vi "Calibration INI tester.vi"() -> ()   [LabVIEW 2020]
uses:
  Typedefs/Calibration config.ctl
  Typedefs/Objective Config.ctl
  Typedefs/Prechirper Cal Config.ctl
  Typedefs/PreChirper constants.ctl
panel:
  in  "Save to":path
  in  "Load from":path
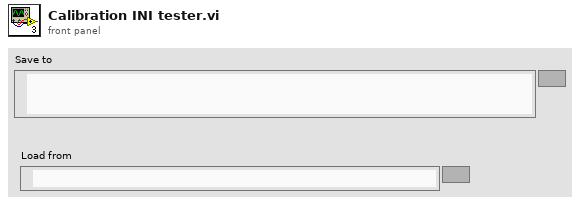
[diagram p1: front panel]
types:
  T1 = typedef "PreChirper constants.ctl" = cluster{"a 1":i32, "b 1":i32, "c 1":i32, "a 2":i32, "b 2":i32, "c 2":i32, "lmin":i32, "lmax":i32}
  T2 = typedef "Prechirper Cal Config.ctl" = cluster{"Wavelength":i32, "Prism 1":i32, "Prism 2":i32}
  T3 = typedef "Objective Config.ctl" = cluster{"Name":string, "Sum X":dbl, "Sum Y":dbl, "Diff X":dbl, "Diff Y":dbl, "Distortion Correction":dbl, "Z_norm to um_scaling":dbl, "X_norm to um_scaling":dbl, "Calibrated Wavelength":dbl}
  T4 = typedef "Calibration config.ctl" = cluster{"Current Objective":string, "Objective Settings":T3[], "PreChirper Values Preset ?":bool, "PreChirper Settings":T2[], "PreChirper Constants":T1}
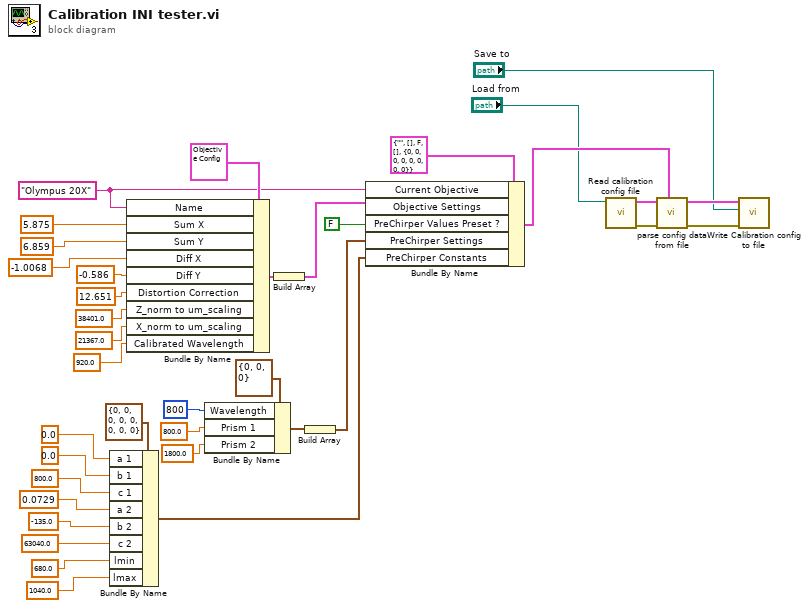
[diagram p0: block diagram]
diagram:
  w35 = "Olympus 20X" ("Current Objective")
  n1 = Bundle By Name(cluster=T1 {"a 1"=0, "b 1"=0, "c 1"=0, "a 2"=0, "b 2"=0, "c 2"=0, "lmin"=0, "lmax"=0} ("Prechirper Constants"), "a 1"=0.0, "b 1"=0.0, "c 1"=800.0, "a 2"=0.0729, "b 2"=-135.0, "c 2"=63040.0, "lmin"=680.0, "lmax"=1040.0) -> (w10:T1)
  n2 = Bundle By Name(cluster=T3 {"Name"="", "Sum X"=0.0, "Sum Y"=0.0, "Diff X"=0.0, "Diff Y"=0.0, "Distortion Correction"=0.0, "Z_norm to um_scaling"=0.0, "X_norm to um_scaling"=0.0, "Calibrated Wavelength"=0.0} ("Objective HW Settings"), "Name"=w35, "Sum X"=5.875, "Sum Y"=6.859, "Diff X"=-1.0068 ("Sum Y"), "Diff Y"=-0.586 ("Sum Y"), "Distortion Correction"=12.651 ("Sum Y"), "Z_norm to um_scaling"=38401.0 ("Sum Y"), "X_norm to um_scaling"=21367.0 ("Sum Y"), "Calibrated Wavelength"=920.0) -> (w26:T3)
  n3 = Bundle By Name(cluster=T2 {"Wavelength"=0, "Prism 1"=0, "Prism 2"=0} ("Prechirper Config"), "Wavelength"=800, "Prism 1"=800.0, "Prism 2"=1800.0) -> (w22:T2)
  n4 = Build Array(w26) -> (w25:T3[])
  n5 = Build Array(w22) -> (w9:T2[])
  n6 = Bundle By Name(cluster=T4 {"Current Objective"="", "Objective Settings"=[], "PreChirper Values Preset ?"=FALSE, "PreChirper Settings"=[], "PreChirper Constants"={"a 1"=0, "b 1"=0, "c 1"=0, "a 2"=0, "b 2"=0, "c 2"=0, "lmin"=0, "lmax"=0}} ("Config cluster IN"), "Current Objective"=w35, "Objective Settings"=w25, "PreChirper Values Preset ?"=FALSE, "PreChirper Settings"=w9, "PreChirper Constants"=w10) -> (w5:T4)
  n7 = call "Read calibration config file.vi"("configuration file path"="Load from") -> ("error out"=w6:errorcluster, "Array"=w7:cluster{"String":string, string[]}[])  [unwired: 9 in]
  n8 = call "parse config data from file.vi"("Calibration Config"=w5, "Error in"=w6, "Array"=w7) -> ("Error out"=w3:errorcluster, "Config cluster"=w2:T4)  [unwired: 7 in]
  n9 = call "Write Calibration config to file.vi"("error in (no error)"=w3, "configuration file path"="Save to", "Calibration config."=w2) -> ()  [unwired: 8 in, 1 out]
